vi "getVoltagesamples.vi"(8 "error in (no error)":errorcluster, 11 "params":refnum<class "JSON Value.lvclass">) -> (0 "error out":errorcluster, 1 "Voltage Samples":dbl[][](array[numeric]), 2 "JSON String":string="cam0", 3 "data":refnum<class "JSON Value.lvclass">)   [LabVIEW 2019]
uses:
  <vilib>/NI/JSON Support for LabVIEW/JSON Value/JSON Value.lvclass
  <vilib>/DAQmx/read.llb/DAQmx Read (Analog 1D DBL 1Chan NSamp).vi
  <vilib>/NI/JSON Support for LabVIEW/JSON Value/Object/Get Value/Get Value (Numeric).vi
  <vilib>/NI/JSON Support for LabVIEW/JSON Value/Object/Get Value/Get Value (String).vi
  <vilib>/DAQmx/create/channels.llb/DAQmx Create Channel (AI-Voltage-Basic).vi
  <vilib>/DAQmx/configure/timing.llb/DAQmx Timing (Sample Clock).vi
  <vilib>/DAQmx/miscellaneous.llb/DAQmx Fill In Error Info.vi
  <vilib>/NI/JSON Support for LabVIEW/JSON Value/New JSON Value/New JSON (Numeric[]).vi
  <vilib>/NI/JSON Support for LabVIEW/JSON Value/New JSON Value/New JSON (Numeric).vi
  <vilib>/NI/JSON Support for LabVIEW/JSON Value/New JSON Value/New JSON ({Value[]}).vi
  <vilib>/NI/NI JSONRPC Server Framework/Classes/Server/JSONRPC Server.lvclass
  <resource>/objmgr/daqmx.rc
panel:
  in  "Vmin":dbl=-0.6
  in  "Vmax":dbl=0.6
  in  "Sample Rate":dbl=1000.0
  in  "Samples":dbl=10.0
  in  "Channel":string="Mod2/ai0"
  in  "Debug":bool
  # "Output Data"
  # "Debug Input Parameters"
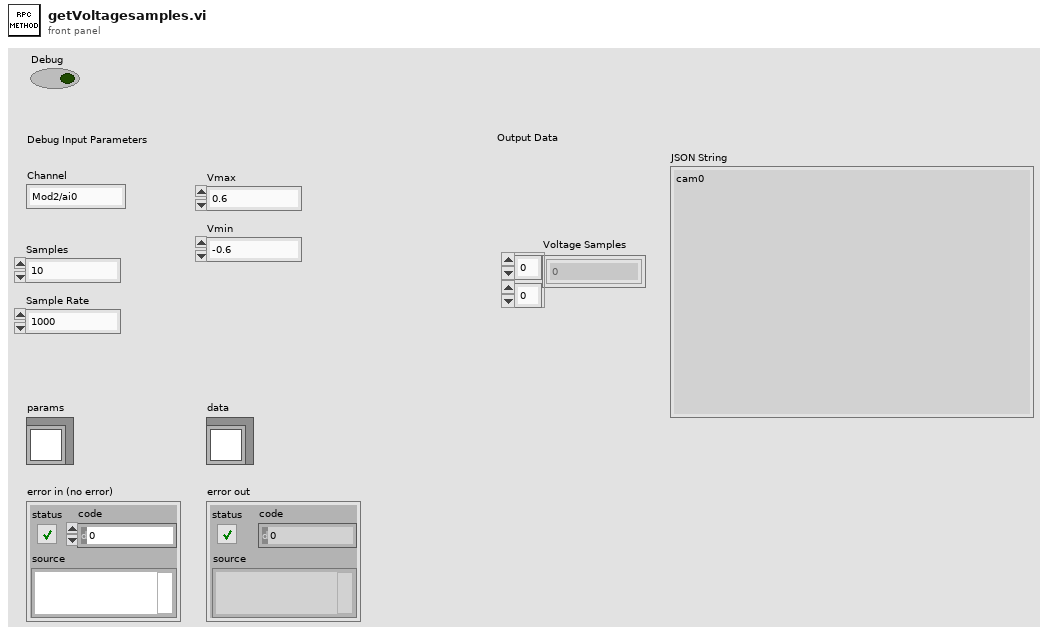
[diagram p1: front panel]
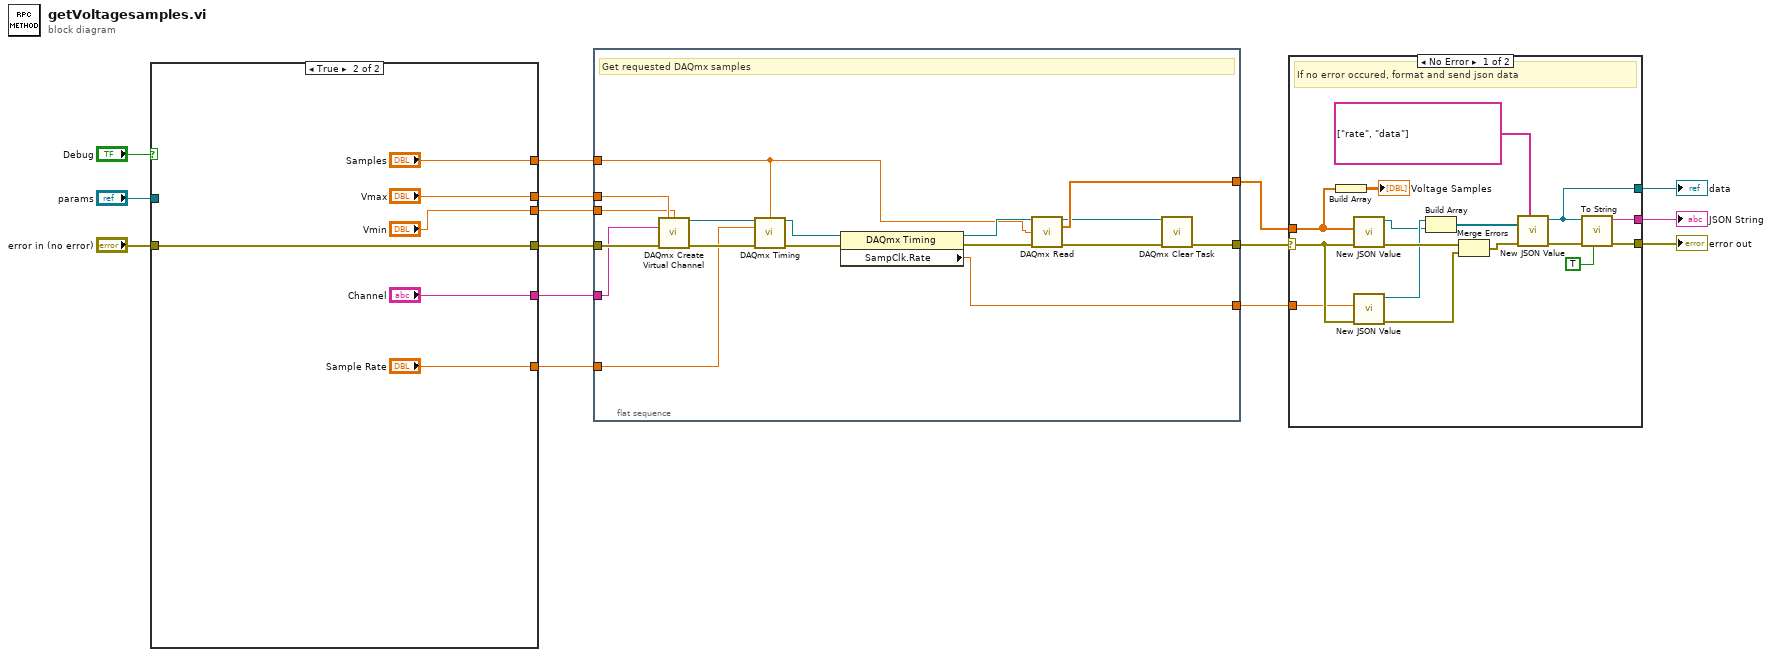
[diagram p0: block diagram]
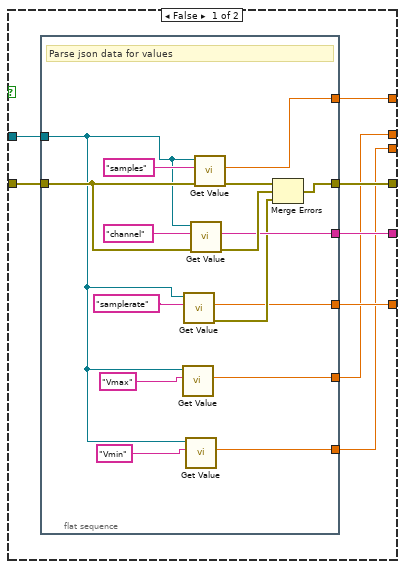
[diagram p2: hidden frame]
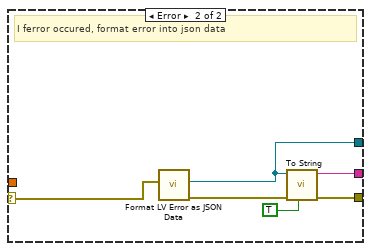
[diagram p3: hidden frame]
diagram:
  n1 = case shown="True" "Debug" {
    tunnel: "params" -> [w23 _]
    tunnel: "error in (no error)" -> [w22 w40]
    tunnel: [w21 w40] -> w13
    tunnel: [w20 "Channel"] -> w8
    tunnel: [w19 "Samples"] -> w7
    tunnel: [w18 "Sample Rate"] -> w5
    tunnel: [w17 "Vmax"] -> w4
    tunnel: [w16 "Vmin"] -> w3
    frame False {
      n2 = flat-sequence {
        tunnel: w23 -> [w28]
        tunnel: w22 -> [w32]
        tunnel: [w36] -> w21
        tunnel: [w34] -> w19
        tunnel: [w33] -> w20
        tunnel: [w29] -> w18
        tunnel: [w25] -> w17
        tunnel: [w24] -> w16
        frame #0 {
          # "Parse json data for values"
          n3 = call-poly <vilib>:"Get Value.vi"("key"="Vmax", "JSON Value in"=w28) -> ("value"=w25:dbl)  [unwired: 8 in, 1 out]
          n4 = call-poly <vilib>:"Get Value.vi"("key"="samplerate", "JSON Value in"=w28) -> ("error out"=w30:errorcluster, "value"=w29:dbl)  [unwired: 8 in]
          n5 = call-poly <vilib>:"Get Value.vi"("key"="Vmin", "JSON Value in"=w28) -> ("value"=w24:dbl)  [unwired: 8 in, 1 out]
          n6 = call-poly <vilib>:"Get Value.vi"("error in (no error)"=w32, "key"="channel", "JSON Value in"=w28) -> ("error out"=w35:errorcluster, "value"=w33:string)  [unwired: 7 in]
          n7 = call-poly <vilib>:"Get Value.vi"("error in (no error)"=w32, "key"="samples", "JSON Value in"=w28) -> ("error out"=w37:errorcluster, "value"=w34:dbl)  [unwired: 7 in]
          n8 = Merge Errors(w37, w35, w30) -> (w36:errorcluster)
        }
      }
    }
    frame True {
    }
  }
  n9 = flat-sequence {
    tunnel: w13 -> [w62]
    tunnel: [w56] -> w10
    tunnel: [w52] -> w9
    tunnel: w8 -> [w61]
    tunnel: w7 -> [w53]
    tunnel: [w49] -> w6
    tunnel: w5 -> [w48]
    tunnel: w4 -> [w47]
    tunnel: w3 -> [w46]
    frame #0 {
      # "Get requested DAQmx samples"
      n10 = call-poly <vilib>:"DAQmx Create Virtual Channel.vi"("maximum value"=w47, "minimum value"=w46, "physical channels"=w61, "error in"=w62) -> ("task out"=w59:refnum<k21>, "error out"=w60:errorcluster)  [unwired: 10 in]
      n11 = call-poly <vilib>:"DAQmx Timing.vi"("task/channels in"=w59, "samples per channel"=w53, "rate"=w48, "error in"=w60) -> ("task out"=w57:refnum<k21>, "error out"=w58:errorcluster)  [unwired: 10 in]
      n12 = property class="DAQmx Timing"(reference=w57, error in=w58) -> (reference out=w54:refnum<k21>, error out=w55:errorcluster, "SampClk.Rate"=w56:dbl)
      n13 = call-poly <vilib>:"DAQmx Read.vi"("task/channels in"=w54, "number of samples per channel"=w53, "error in"=w55) -> ("task out"=w50:refnum<k21>, "data"=w52:dbl[], "error out"=w51:errorcluster)  [unwired: 10 in]
      n14 = call <vilib>:"DAQmx Clear Task.vi"("task in"=w50, "error in"=w51) -> ("error out"=w49:errorcluster)  [unwired: 13 in]
    }
  }
  n15 = case shown="No Error" w6 {
    selector: w6 -> [w75 w84]
    tunnel: [w70 w81] -> w12
    tunnel: [w69 w82] -> w11
    tunnel: w9 -> [w65 _]
    tunnel: w10 -> [w72 _]
    tunnel: [w67 w79] -> w2
    frame No Error {
      # "If no error occured, format and send json data"
      n16 = Build Array(w65) -> (→"Voltage Samples":dbl[][])
      n17 = call-poly <vilib>:"New JSON Value.vi"("error in (no error)"=w75, "Numeric Array"=w65) -> ("error out"=w78:errorcluster, "JSON Value out"=w63:refnum<class "JSON Value.lvclass">)  [unwired: 8 in]
      n18 = call-poly <vilib>:"New JSON Value.vi"("error in (no error)"=w75, "value"=w72) -> ("error out"=w76:errorcluster, "JSON Value out"=w64:refnum<class "JSON Value.lvclass">)  [unwired: 8 in]
      n19 = Build Array(w64, w63) -> (w74:refnum<class "JSON Value.lvclass">[])
      n20 = Merge Errors(w78, w76) -> (w77:errorcluster)
      n21 = call-poly <vilib>:"New JSON Value.vi"("keys"=string[] ["rate", "data"], "error in (no error)"=w77, "values"=w74) -> ("error out"=w71:errorcluster, "JSON Value out"=w69:refnum<class "JSON Value.lvclass">)  [unwired: 7 in]
      n22 = call <vilib>:"To String.vi"("pretty print? (F)"=TRUE, "error in (no error)"=w71, "JSON Value in"=w69) -> ("error out"=w70:errorcluster, "String"=w67:string)  [unwired: 7 in]
    }
    frame Error {
      # "I ferror occured, format error into json data"
      n23 = call <vilib>:"Format LV Error as JSON Data.vi"("error in"=w84) -> ("error out"=w83:errorcluster, "Error Value out"=w82:refnum<class "JSON Value.lvclass">)  [unwired: 9 in]
      n24 = call <vilib>:"To String.vi"("pretty print? (F)"=TRUE, "error in (no error)"=w83, "JSON Value in"=w82) -> ("error out"=w81:errorcluster, "String"=w79:string)  [unwired: 7 in]
    }
  }
  "data" <- w11
  "error out" <- w12
  "JSON String" <- w2
